vi "execute.vi"(8 "error in (no error)":errorcluster, 9 "data collection in":refnum<class "GenericComponent.lvclass">, 10 "imaging mode in":refnum<class "GenericComponent.lvclass">, 11 "adapter in":refnum<class "AdapterTS090827ImagingModeToDataCollection.lvclass">) -> (0 "error out":errorcluster, 1 "data collection out":refnum<class "GenericComponent.lvclass">, 2 "imaging mode out":refnum<class "GenericComponent.lvclass">, 3 "adapter out":refnum<class "AdapterTS090827ImagingModeToDataCollection.lvclass">)   [LabVIEW 2010, in "AdapterTS090827ImagingModeToDataCollection.lvclass"]
uses:
  AdapterTS090827ImagingModeToDataCollection.lvclass
  common/classes/GenericComponent/GenericComponent/GenericComponent.lvclass
  DataCollection/DataCollectionDL090215/DataCollectionDL090215/DataCollectionDL090215.lvclass
  ImagingMode/ImagingModeTS090821Circular2D/ImagingModeTS090821Circular2D/ImagingModeTS090821Circular2D.lvclass
panel:
  # "imaging mode: ImagingModeTS090821Circular2D\ndata collection: DataCollectionDL090215"
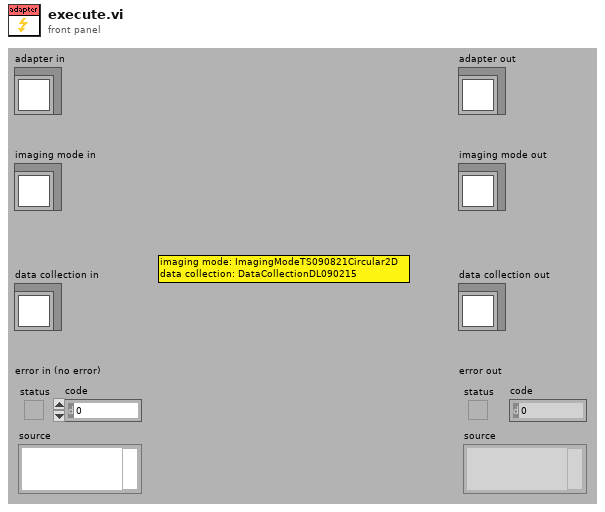
[diagram p1: front panel]
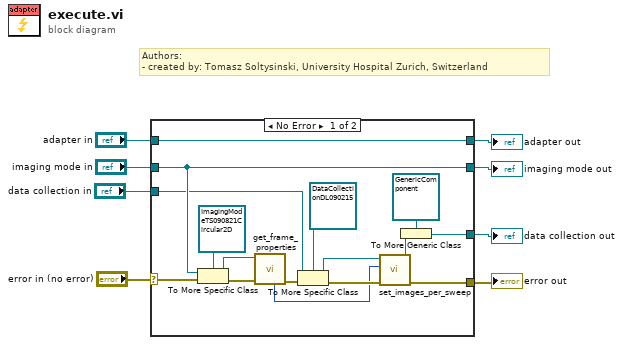
[diagram p0: block diagram]
diagram:
  # "Authors: \n- created by: Tomasz Soltysinski, University Hospital Zurich, Switzerland"
  n1 = case shown="No Error" "error in (no error)" {
    selector: "error in (no error)" -> [w23 w28]
    tunnel: [w24 w27] -> w6
    tunnel: "adapter in" -> [w24 w27]
    tunnel: [w22 w26] -> w4
    tunnel: "imaging mode in" -> [w22 w26]
    tunnel: [w20 w25] -> w3
    tunnel: "data collection in" -> [w19 w25]
    tunnel: [w13 w28] -> w1
    frame No Error {
      n2 = To More Specific Class(target class=refnum<class "ImagingModeTS090821Circular2D.lvclass"> refnum ("ImagingModeTS090821Circular2D.lvclass"), reference=w22, error in=w23) -> (specific class reference=w11:refnum<class "ImagingModeTS090821Circular2D.lvclass">, error out=w18:errorcluster)
      n3 = call-dynamic "get_frame_properties.vi"("error in (no error)"=w18, "ScanModeTS090821Circular2D in"=w11) -> ("error out"=w17:errorcluster, "number of frames"=w14:i32)  [unwired: 5 in, 3 out]
      n4 = To More Specific Class(target class=refnum<class "DataCollectionDL090215.lvclass"> refnum ("DataCollectionDL090215.lvclass"), reference=w19, error in=w17) -> (specific class reference=w10:refnum<class "DataCollectionDL090215.lvclass">, error out=w15:errorcluster)
      n5 = call-dynamic "set_images_per_sweep.vi"("error in (no error)"=w15, "images per sweep"=w14, "DL090215DataCollection.lvclass in"=w10) -> ("error out"=w13:errorcluster, "DL090215DataCollection.lvclass out"=w12:refnum<class "DataCollectionDL090215.lvclass">)  [unwired: 7 in]
      n6 = To More Generic Class(target class=refnum<class "GenericComponent.lvclass"> refnum ("GenericComponent.lvclass"), reference=w12) -> (generic class reference=w20:refnum<class "GenericComponent.lvclass">)
    }
    frame Error {
    }
  }
  "error out" <- w1
  "adapter out" <- w6
  "imaging mode out" <- w4
  "data collection out" <- w3
